vi "Exportar a Excel.vi"(7 "Nombre Equipo":string="Generador", 8 "error in (no error)":errorcluster, 11 "Data":dbl[][](array[numeric])) -> (0 "error out":errorcluster)   [LabVIEW 2018]
uses:
  <vilib>/Utility/NIReport.llb/Report Type.ctl
  <vilib>/addons/_office/excel.llb/Excel Easy Table (num).vi
  <vilib>/Utility/NIReport.llb/NI_report.lvclass
  <vilib>/Utility/NIReport.llb/Excel/NI_Excel.lvclass
  <vilib>/Utility/NIReport.llb/NI_ReportGenerationCore.lvlib
  <vilib>/addons/_office/NI_ReportGenerationToolkit.lvlib
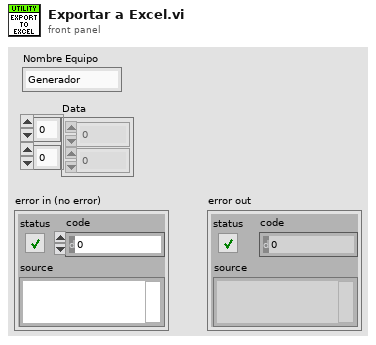
[diagram p1: front panel]
types:
  T1 = typedef "NI_ReportGenerationCore.lvlib/Report Type.ctl" = enum16{"HTML", "Word", "Excel"}
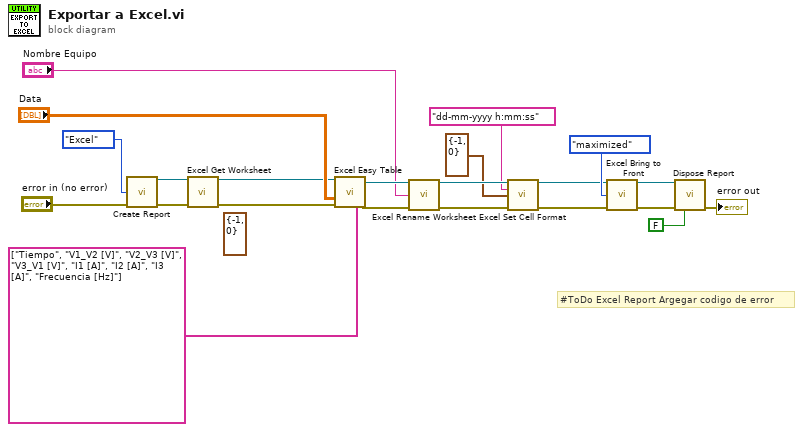
[diagram p0: block diagram]
diagram:
  (unwired) cluster{"row":i32, "column":i32} {"row"=-1, "column"=0} ("start (-1, -1)")
  # "#ToDo Excel Report Argegar codigo de error"
  n1 = call <vilib>:"Create Report.vi"("report type"=Report_Type."Excel" ("Report Type"), "error in (no error)"="error in (no error)") -> ("report out"=w11:refnum<class "NI_report.lvclass">, "error out"=w15:errorcluster)  [unwired: 12 in]
  n2 = call <vilib>:"Excel Get Worksheet.vi"("report in"=w11, "error in (no error)"=w15) -> ("report out"=w6:refnum<class "NI_report.lvclass">, "error out"=w12:errorcluster)  [unwired: 12 in]
  n3 = call-poly <vilib>:"Excel Easy Table.vi"("report in"=w6, "text data"="Data", "error in (no error)"=w12, "column headers"=string[] ["Tiempo", "V1_V2 [V]", "V2_V3 [V]", "V3_V1 [V]", "I1 [A]", "I2 [A]", "I3 [A]", "Frecuencia [Hz]"]) -> ("report out"=w10:refnum<class "NI_report.lvclass">, "error out"=w9:errorcluster)  [unwired: 7 in, 3 out]
  n4 = call <vilib>:"Excel Rename Worksheet.vi"("report in"=w10, "worksheet name (\"\")"="Nombre Equipo", "error in (no error)"=w9) -> ("report out"=w4:refnum<class "NI_report.lvclass">, "error out"=w8:errorcluster)  [unwired: 11 in]
  n5 = call <vilib>:"Excel Set Cell Format.vi"("report in"=w4, "number format"="dd-mm-yyyy h:mm:ss", "start (-1, -1)"=cluster{"row":i32, "column":i32} {"row"=-1, "column"=0}, "error in (no error)"=w8) -> ("report out"=w3:refnum<class "NI_report.lvclass">, "error out"=w5:errorcluster)  [unwired: 10 in]
  n6 = call <vilib>:"Excel Bring to Front.vi"("report in"=w3, "window state (maximized)"=enum16{"maximized", "minimized", "normal"}."maximized", "error in (no error)"=w5) -> ("report out"=w18:refnum<class "NI_report.lvclass">, "error out"=w17:errorcluster)  [unwired: 11 in]
  n7 = call-dynamic "Dispose Report.vi"("report in"=w18, "error in (no error)"=w17, "close report? (T)"=FALSE ("Close Report? (T)")) -> ("error out"=→"error out":errorcluster)  [unwired: 12 in]
